vi "Convert Dbl to ALtitude.vi"(11 "Setpoint":sgl) -> (3 "Altitude Out":T1)   [LabVIEW 2013]
doc: "Converts a number to something that fits in the ALT SET control."
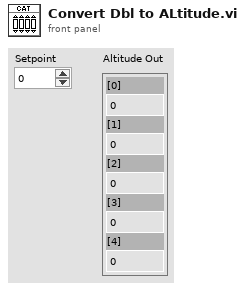
[diagram p1: front panel]
types:
  T1 = cluster{"[0]":i8, "[1]":i8, "[2]":i8, "[3]":i8, "[4]":i8}
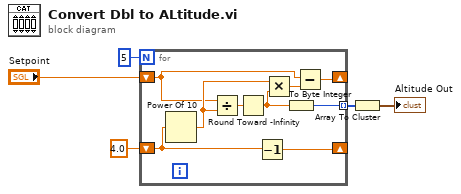
[diagram p0: block diagram]
diagram:
  n1 = for {
    N: 5 -> [_]
    shift-right: [w6] -> _
    shift-left: "Setpoint" -> [w7]
    tunnel: [w13] -> w3 mode=indexing
    shift-right: [w12] -> _
    shift-left: 4.0 -> [w11]
    n2 = Power Of 10(x=w11) -> (10^x=w9:dbl)
    n3 = Divide(x=w7, y=w9) -> (x/y=w14:dbl)
    n4 = Round Toward -Infinity(1:w14) -> (0:w10:dbl)
    n5 = Decrement(x=w11) -> (x-1=w12:dbl)
    n6 = Multiply(x=w9, y=w10) -> (x*y=w8:dbl)
    n7 = To Byte Integer(number=w10) -> (8bit integer=w13:i8)
    n8 = Subtract(x=w7, y=w8) -> (x-y=w6:dbl)
  }
  n9 = Array To Cluster(array=w3) -> (cluster=→"Altitude Out":T1)
